vi "Remove Empty Sections .vi"(11 "Array in":refnum<class "Section.lvclass">[](array[class])) -> (3 "Array out":refnum<class "Section.lvclass">[](array[class]))   [LabVIEW 2021, in "TAF Proj Document Type.lvlib" / "TAF Proj.lvclass"]
uses:
  <vilib>/Wovalab/AntiDoc/Document Type/Add-ons/LabVIEW TAF Project/TAF Proj/TAF Proj.lvclass
  <vilib>/Wovalab/AntiDoc/Section/Section.lvclass
  <vilib>/Wovalab/AntiDoc/Sub Section/Sub Section.lvclass
  C:/Program Files (x86)/National Instruments/LabVIEW 2021/vi.lib/Wovalab/AntiDoc/Section/Section.lvclass
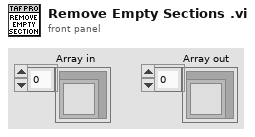
[diagram p1: front panel]
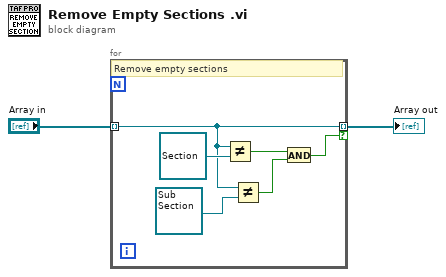
[diagram p0: block diagram]
diagram:
  n1 = for {
    tunnel: "Array in" -> [w6] mode=indexing
    tunnel: [w6] -> w2 mode=indexing if=w4
    # "Remove empty sections"
    n2 = Not Equal?(x=w6, y=refnum<class "Section.lvclass"> refnum ("Section out")) -> (x != y?=w7:bool)
    n3 = Not Equal?(x=w6, y=refnum<class "Sub Section.lvclass"> refnum ("Antidoc:Sub Section")) -> (x != y?=w3:bool)
    n4 = And(x=w7, y=w3) -> (x .and. y?=w4:bool)
  }
  "Array out" <- w2
